vi "DecodeCommands.vi"(1 "element":u8[](array[numeric]), 3 "Key":i32=-1, 5 "error in (no error)":errorcluster) -> (14 "Commands":T1(array[cluster]), 15 "element 2":u8[](array[numeric]), 19 "error out":errorcluster)   [LabVIEW 2023, in "Referee.lvclass"]
uses:
  Referee.lvclass
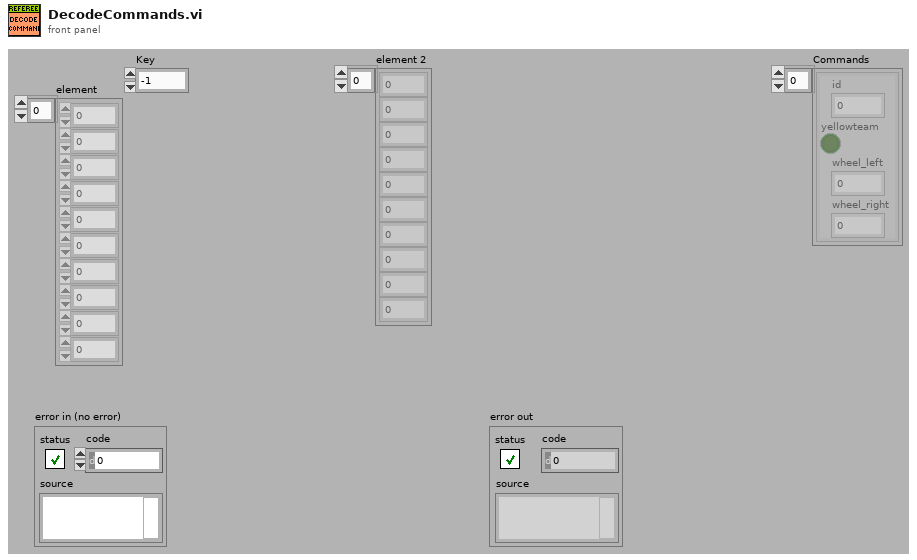
[diagram p1: front panel]
types:
  T1 = cluster{"id":dbl, "yellowteam":bool, "wheel_left":dbl, "wheel_right":dbl}[]
  T2 = cluster{"id":dbl, "yellowteam":bool, "wheel_left":dbl, "wheel_right":dbl}
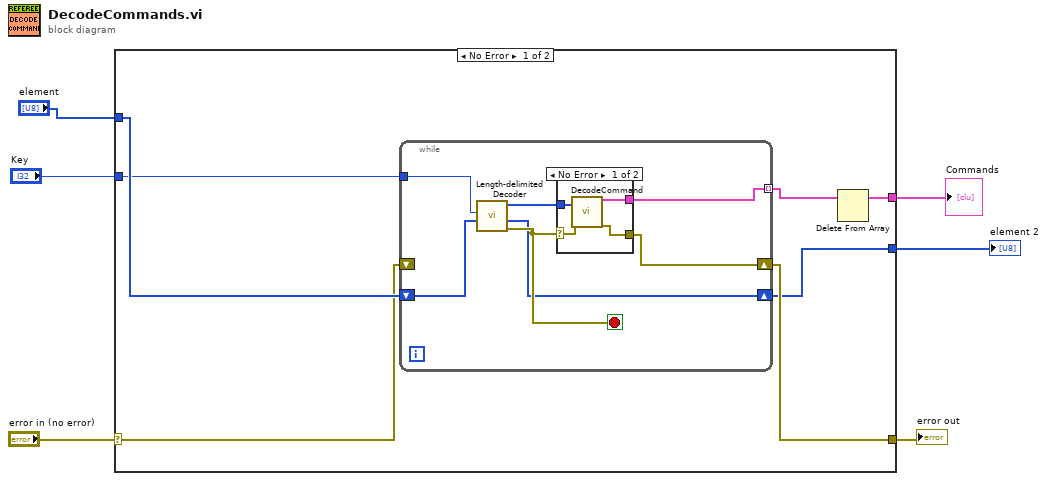
[diagram p0: block diagram]
diagram:
  n1 = case shown="No Error" "error in (no error)" {
    selector: "error in (no error)" -> [w10 w25]
    tunnel: [w9 w25] -> w5
    tunnel: [w7 _] -> w4
    tunnel: "element" -> [w12 _]
    tunnel: "Key" -> [w11 _]
    tunnel: [w8 _] -> w1
    frame No Error {
      n2 = while {
        tunnel: w11 -> [w18]
        shift-right: [w13] -> w7
        shift-left: w12 -> [w19]
        tunnel: [w17] -> w8 mode=indexing
        shift-right: [w15] -> w9
        shift-left: w10 -> [_]
        stop <- w16 stop-if-true
        n3 = call "Length-delimited Decoder.vi"("Array"=w19, "Key"=w18) -> ("error out"=w16:errorcluster, "array w/ subset deleted"=w13:u8[], "Length-delimited"=w14:u8[])  [unwired: 6 in, 1 out]
        n4 = case shown="No Error" w16 {
          selector: w16 -> [w21 w24]
          tunnel: w14 -> [w23 _]
          tunnel: [w22 _] -> w17
          tunnel: [w20 w24] -> w15
          frame No Error {
            n5 = call "DecodeCommand.vi"("element"=w23, "error in (no error)"=w21) -> ("Command"=w22:T2, "error out"=w20:errorcluster)  [unwired: 16 in]
          }
          frame Error {
          }
        }
      }
      n6 = Delete From Array(array=w8) -> ()  [unwired: 2 in, 2 out]
    }
    frame Error {
    }
  }
  "error out" <- w5
  "element 2" <- w4
  "Commands" <- w1
